vi "CreateCommand.vi"(8 "error in (no error)":errorcluster, 9 "param":variant, 10 "Command":T1, 11 "CommandFactory in":refnum<class "CommandFactory.lvclass">) -> (0 "error out":errorcluster, 2 "Command.lvclass":refnum<class "Command.lvclass">, 3 "CommandFactory out":refnum<class "CommandFactory.lvclass">)   [LabVIEW 2020, in "CommandFactory.lvclass"]
uses:
  CommandFactory.lvclass
  commandList.ctl
  Command/Command.lvclass
  ChangeSlitWidth/ChangeSlitWidth.lvclass
  C:/Users/Eric Coughlin/repos/ss_monochromator/WindowsController/Commands/Command/Command.lvclass
  Typedefs/slit.ctl
  Typedefs/SlitType.ctl
  Typedefs/slitWidth.ctl
  ChangeSlitWidth/ChangeSlitWidth.lvclass/ChangeSlitWidth.ctl
  ChangeWavelength/ChangeWavelength.lvclass
  Typedefs/wavelength.ctl
  ChangeWavelength/ChangeWavelength.lvclass/ChangeWavelength.ctl
  SelectGrating/SelectGrating.lvclass
  Typedefs/GratingType.ctl
  SelectGrating/SelectGrating.lvclass/SelectGrating.ctl
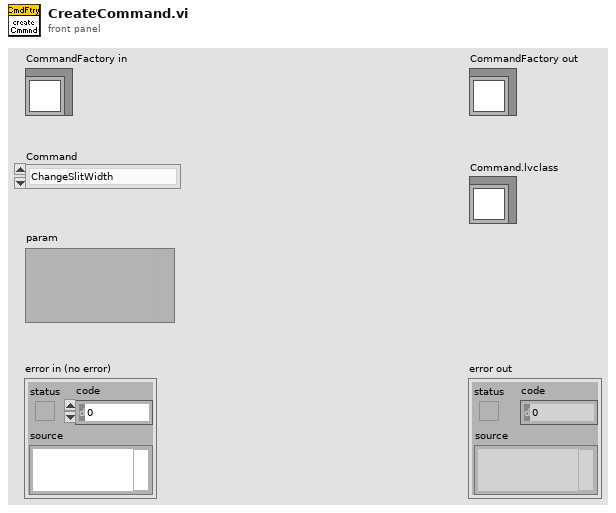
[diagram p1: front panel]
types:
  T1 = typedef "commandList.ctl" = enum16{"ChangeSlitWidth", "ChangeWavelendth", "SelectGrating"}
  T2 = typedef "slit.ctl" = cluster{"SlitType":T3, "Width":T4}
  T3 = typedef "SlitType.ctl" = enum16{"Front Entrance", "Side Entrance", "Front Exit", "Side Exit", "First Intermediate", "Second Intermediate"}
  T4 = typedef "slitWidth.ctl" = dbl
  T5 = typedef "wavelength.ctl" = dbl
  T6 = typedef "GratingType.ctl" = enum16{"Blue", "Red", "Mirror"}
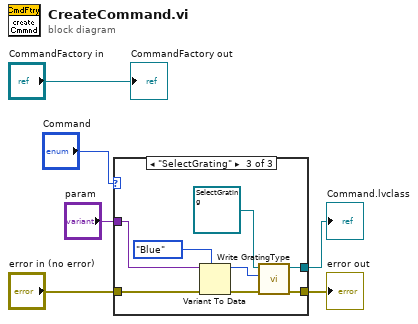
[diagram p0: block diagram]
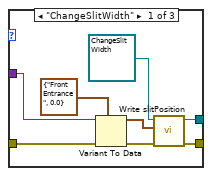
[diagram p2: hidden frame]
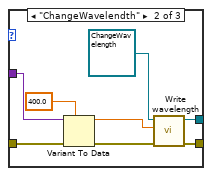
[diagram p3: hidden frame]
diagram:
  n1 = case shown="\"SelectGrating\"" "Command" {
    tunnel: "error in (no error)" -> [w12 w20 w26]
    tunnel: [w8 w15 w24] -> w4
    tunnel: "param" -> [w13 w21 w27]
    tunnel: [w7 w16 w25] -> w1
    frame "ChangeSlitWidth" {
      n2 = Variant To Data(error in=w12, type=T2 {"SlitType"=enum."Front Entrance", "Width"=0.0} ("slitPosition"), Variant=w13) -> (data=w10:T2, error out=w9:errorcluster)
      n3 = call "Write slitPosition.vi"("error in (no error)"=w9, "slitPosition"=w10, "ChangeSlitWidth in"=refnum<class "ChangeSlitWidth.lvclass"> refnum ("ChangeSlitWidth.lvclass")) -> ("error out"=w8:errorcluster, "ChangeSlitWidth out"=w7:refnum<class "ChangeSlitWidth.lvclass">)  [unwired: 7 in]
    }
    frame "ChangeWavelendth" {
      n4 = Variant To Data(error in=w20, type=T5 400.0 ("wavelength"), Variant=w21) -> (data=w18:T5, error out=w19:errorcluster)
      n5 = call "Write wavelength.vi"("error in (no error)"=w19, "wavelength"=w18, "ChangeWavelength in"=refnum<class "ChangeWavelength.lvclass"> refnum ("ChangeWavelength.lvclass")) -> ("error out"=w15:errorcluster, "ChangeWavelength out"=w16:refnum<class "ChangeWavelength.lvclass">)  [unwired: 7 in]
    }
    frame "SelectGrating" {
      n6 = Variant To Data(error in=w26, type=GratingType."Blue" ("GratingType"), Variant=w27) -> (data=w28:T6, error out=w23:errorcluster)
      n7 = call "Write GratingType.vi"("error in (no error)"=w23, "GratingType"=w28, "SelectGrating in"=refnum<class "SelectGrating.lvclass"> refnum ("SelectGrating.lvclass")) -> ("error out"=w24:errorcluster, "SelectGrating out"=w25:refnum<class "SelectGrating.lvclass">)  [unwired: 7 in]
    }
  }
  "error out" <- w4
  "Command.lvclass" <- w1
  "CommandFactory out" <- "CommandFactory in"
